vi "ClearWfrm.vi"(8 "ErrorArray In":errorcluster[](array[cluster]), 10 "clFrontPanelControlRefs":T1, 11 "NISTBus In":refnum<class "NISTBus.lvclass">) -> (0 "ErrorArray Out":errorcluster[](array[cluster]), 3 "NISTBus Out":refnum<class "NISTBus.lvclass">)   [LabVIEW 2014, in "Bus.lvlib" / "NISTBus.lvclass"]
uses:
  NISTBus.lvclass
  Framework/FrontPanel/TypeDefs/clFrontPanelControlRefs.ctl
  FGenPlugins/MyPluginBaseClass/TypeDef/PluginParams.ctl
  WfrmGenerator/WfrmPlugins/EventPluginBaseClass/TypeDefs/dblEvtSignalArray.ctl
  FGenPlugins/MyPluginBaseClass/TypeDef/CreateArbWfrmParams.ctl
  WfrmGenerator/WfrmPlugins/EventPluginBaseClass/TypeDefs/clEvtConfig.ctl
  WfrmGenerator/WfrmModule/PublicAPI/Arguments/Requests/dblEvtParams.ctl
  FGenPlugins/MyPluginBaseClass/TypeDef/ConfigArbWfrmParams.ctl
  FGenPlugins/MyPluginBaseClass/TypeDef/TriggerParams.ctl
  <userlib>/NIST/NISTErrorLib/NISTErrorLib.lvlib
  FGenPlugins/MyPluginBaseClass/NISTFGenPluginsBase.lvclass
  WfrmGenerator/WfrmPlugins/EventPluginBaseClass/BaseWfrmPlugin.lvclass
  Framework/TestFramework.lvlib
  WfrmGenerator/WfrmModule/WfrmModule.lvlib
panel:
  # "When you add a control \non the front panel, add a\nreference for it in this\ntype def.  This cluster\nwill hold all of the refer-\nences to the front panel\ncontrols in order to pass\nthese control references \nto subvis."
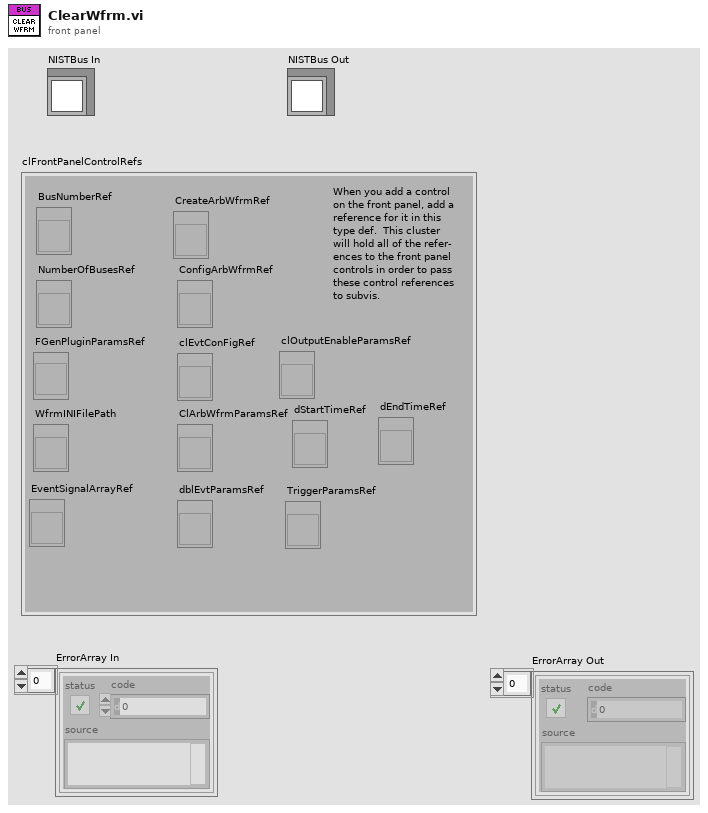
[diagram p1: front panel]
types:
  T1 = typedef "TestFramework.lvlib/clFrontPanelControlRefs.ctl" = cluster{"BusNumberRef":refnum<vi>, "NumberOfBusesRef":refnum<vi>, "FGenPluginParamsRef":refnum<vi>, "WfrmINIFilePath":refnum<vi>, "EventSignalArrayRef":refnum<vi>, "CreateArbWfrmRef":refnum<vi>, "clEvtConFigRef":refnum<vi>, "dblEvtParamsRef":refnum<vi>, "clOutputEnableParamsRef":refnum<vi>, "ConfigArbWfrmRef":refnum<vi>, "ClArbWfrmParamsRef":refnum<vi>, "dStartTimeRef":refnum<vi>, "dEndTimeRef":refnum<vi>, "TriggerParamsRef":refnum<vi>}
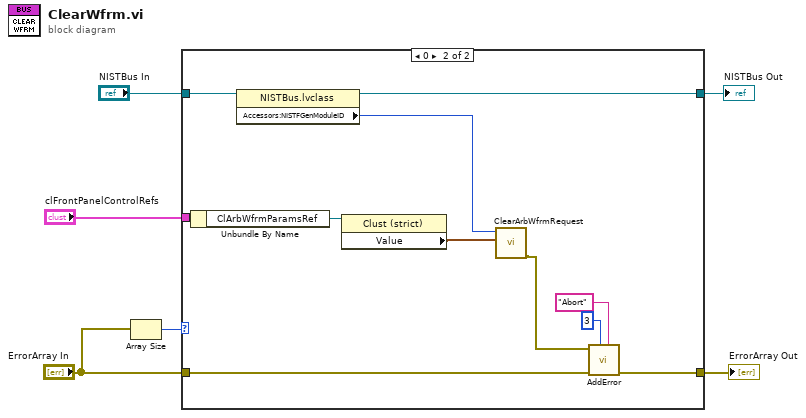
[diagram p0: block diagram]
diagram:
  n1 = Array Size(array="ErrorArray In") -> (size(s)=w6:i32)
  n2 = case shown="0" w6 {
    tunnel: "ErrorArray In" -> [w8 w17]
    tunnel: [w8 w16] -> w4
    tunnel: [w7 w14] -> w3
    tunnel: "NISTBus In" -> [w7 w15]
    tunnel: "clFrontPanelControlRefs" -> [_ w13]
    frame 1, Default {
    }
    frame 0 {
      n3 = Unbundle By Name(w13) -> ("ClArbWfrmParamsRef"=w12:refnum<vi>)
      n4 = property class="NISTBus.lvclass"(reference=w15) -> (reference out=w14:refnum<class "NISTBus.lvclass">, "Accessors:NISTFGenModuleID"=w11:i32)  [unwired: 1 in, 1 out]
      n5 = property class="Clust (strict)"(reference=w12) -> ("Value"=w9:cluster{"iIndex":i32})  [unwired: 1 in, 2 out]
      n6 = call "ClearArbWfrmRequest.vi"("ClrArbWfrmParams"=w9, "ModuleID"=w11) -> ("error out"=w10:errorcluster)  [unwired: 9 in]
      n7 = call <userlib>:"AddError.vi"("Severity"="Abort" ("String"), "Priority"=u8 3, "ErrorArray"=w17, "error in (no error)"=w10) -> ("ErrorArray"=w16:errorcluster[])  [unwired: 6 in, 1 out]
    }
  }
  "NISTBus Out" <- w3
  "ErrorArray Out" <- w4
